vi "DevB.Set Phase.vi"(8 "error in (no error)":errorcluster, 10 "Phase":i32, 11 "DevB Session in":T1) -> (0 "error out":errorcluster, 3 "DevB Session out":T1)   [LabVIEW 2018]
uses:
  typedefs/DevB.Session.ctl
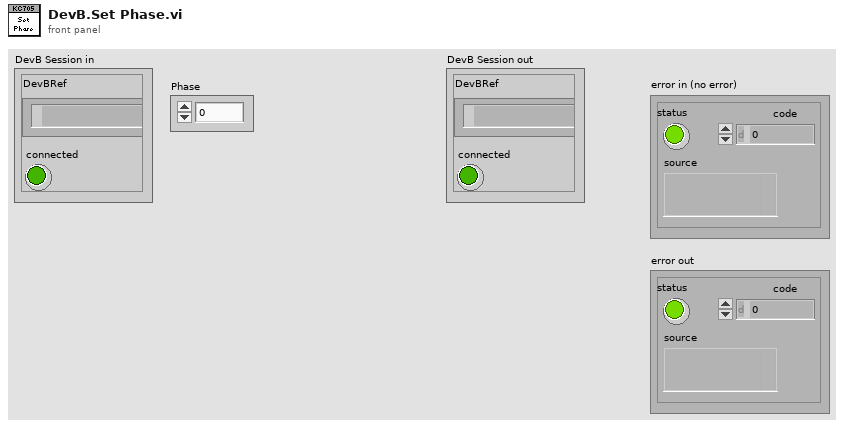
[diagram p1: front panel]
types:
  T1 = typedef "DevB.Session.ctl" = cluster{"DevBRef":refnum<visa-resource-name>, "connected":bool}
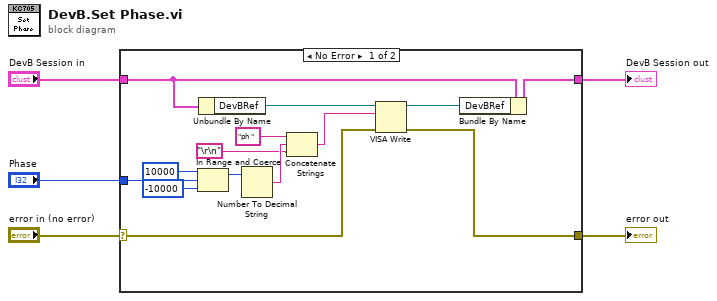
[diagram p0: block diagram]
diagram:
  n1 = case shown="No Error" "error in (no error)" {
    selector: "error in (no error)" -> [w16 w21]
    tunnel: "DevB Session in" -> [w18 w20]
    tunnel: [w15 w21] -> w3
    tunnel: [w14 w20] -> w2
    tunnel: "Phase" -> [w12 _]
    frame No Error {
      n2 = In Range and Coerce(upper limit=10000, x=w12, lower limit=-10000) -> (coerced(x)=w9:i32)  [unwired: 1 out]
      n3 = Unbundle By Name(w18) -> ("DevBRef"=w19:refnum<visa-resource-name>)
      n4 = Number To Decimal String(number=w9) -> (decimal integer string=w8:string)  [unwired: 1 in]
      n5 = Concatenate Strings("ph ", w8, "\r\n") -> (w7:string)
      n6 = VISA Write(VISA resource name=w19, write buffer=w7, error in (no error)=w16) -> (VISA resource name out=w17:refnum<visa-resource-name>, error out=w15:errorcluster)  [unwired: 1 out]
      n7 = Bundle By Name(cluster=w18, "DevBRef"=w17) -> (w14:T1)
    }
    frame Error {
    }
  }
  "DevB Session out" <- w2
  "error out" <- w3
